vi "VisionNetworkingGlobal.vi"() -> ()   [LabVIEW 2023]
panel:
  in  "Vision/RightTime":dbl
  in  "Vision/RightAngle":dbl
  in  "Vision/RightY":dbl
  in  "Vision/RightX":dbl
  in  "Vision/LeftTime":dbl
  in  "Vision/LeftAngle":dbl
  in  "Vision/LeftY":dbl
  in  "Vision/LeftX":dbl
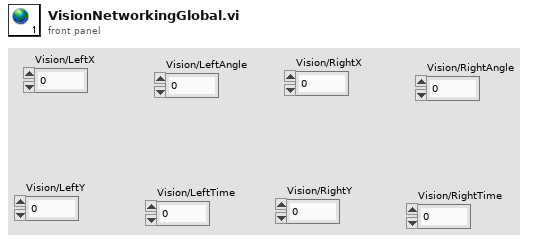
[diagram p1: front panel]
diagram:
